vi "getDesiredFM.vi"(8 "frac":dbl[](array[numeric]), 10 "eC":bool[](array[boolean]), 11 "W":dbl) -> (3 "FM":dbl[](array[numeric]))   [LabVIEW 2024]
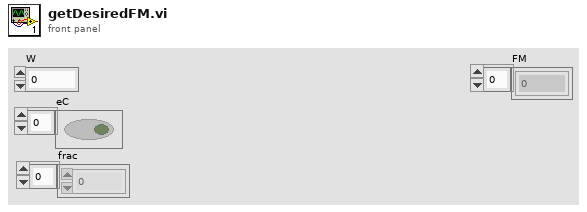
[diagram p1: front panel]
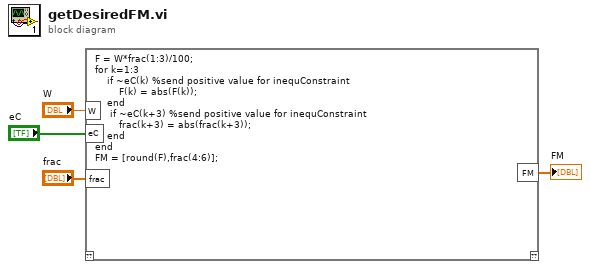
[diagram p0: block diagram]
diagram:
  n1 = mathscript code="F = W*frac(1:3)/100;\nfor k=1:3\n    if ~eC(k) %send positive value for inequConstraint\n        F(k) = abs(F(k));\n    end\n     if ~eC(k+3) %send positive value for inequConstraint\n        frac(k+3) = abs(frac(k+3));\n    end\nend\nFM = [round(F),frac(4:6)];"("W"="W", "frac"="frac", "eC"="eC") -> ("FM"=→"FM":dbl[])  [unwired: 1 in, 1 out]
